vi "Balance Wheel.vi"() -> ()   [LabVIEW 2016]
uses:
  <vilib>/userdefined/High Color/nirio_resource_hc.ctl
  <vilib>/FPGAPlugInAG/myRIO-1900/niLvFpga_Open_myRIO-1900.vi
  <vilib>/rvi/interface/common/dynamic/niFpgaDynamicAddResources.vi
  <vilib>/Utility/error.llb/Error Cluster From Error Code.vi
  <vilib>/rvi/errors/niLvFpgaAdjustHostInterfaceError.vi
  <vilib>/FPGAPlugInAG/Dynamic/niLvFpga_Close_Dynamic.vi
  <vilib>/rvi/interface/nirviOpenFPGA/nirviOpenFPGA.xnode
  FPGA Bitfiles/BalanceWheel_FPGATarget_QuadratureEncode_czObzEe7hTA.lvbitx
  Quadrature Encoder FPGA.vi
  <vilib>/rvi/interface/nirviReadWriteControl/nirviReadWriteControl.xnode
  <vilib>/rvi/interface/nirviCloseFPGA/nirviCloseFPGA.xnode
  <vilib>/rvi/interface/Simulation/niFpgaSimulationCallBeginRW.vi
  NiFpgaLv.dll
panel:
  out "left":dbl=-0.003427734375000213 format="%#.1f"
  out "Rght":dbl=-0.003427734375000213 format="%#.1f"
  out "Desired Left Wheel Speed":dbl(knob)=-8.054739050568652e-09 scale=-5.0..5.0
  out "Displacement":dbl=0.9789672851562501
  out "Encoder Position 2":i32=45332
  in  "resource name":T1="RIO0"
  out "Encoder Position 1":i32=34865
  out "Right Wheel Speed":dbl(knob)=0.00244140625 scale=-5.0..5.0
  out "Left Wheel Speed":dbl(knob) scale=-5.0..5.0
  out "Speed of Car":dbl(knob)=0.001220703125 scale=-5.0..5.0
  out "Desired Right Wheel Speed":dbl(knob)=-8.054739050568652e-09 scale=-5.0..5.0
  out "Desired Speed of Car":dbl(knob)=-8.054739050568652e-09 scale=-5.0..5.0
  out "PID Right Wheel":dbl(knob)=0.20910621206179827 scale=-10.0..10.0
  out "PID Left Wheel":dbl(knob)=0.21032691478406132 scale=-10.0..10.0
  in  "KI (Right)":dbl=0.001
  in  "KP (Right)":dbl=0.5
  in  "KD (Right)":dbl
  in  "KI (Left)":dbl=0.001
  in  "KP (Left)":dbl=0.5
  in  "KD (Left)":dbl
  in  "stop":bool
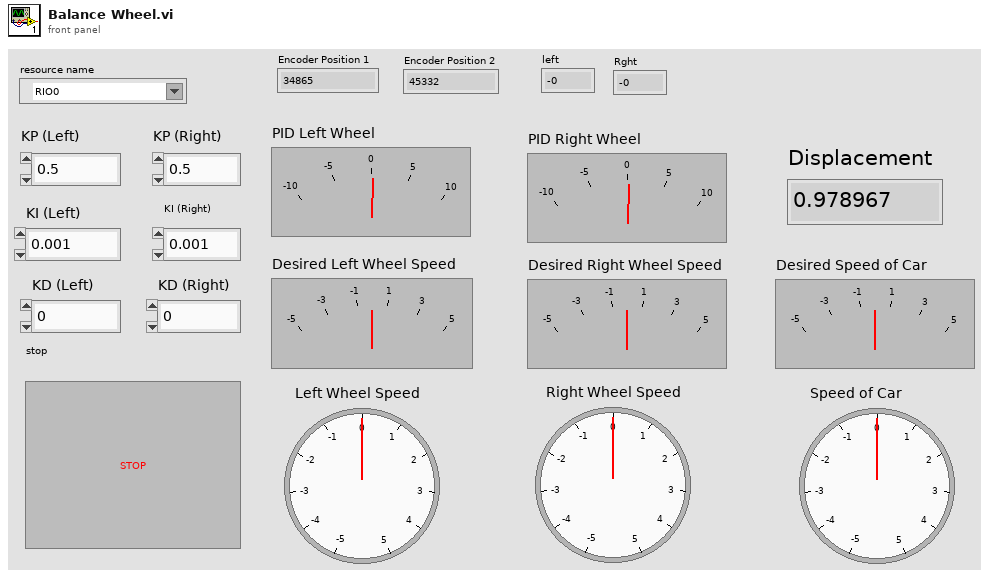
[diagram p1: front panel]
types:
  T1 = typedef "nirio_resource_hc.ctl" = tag
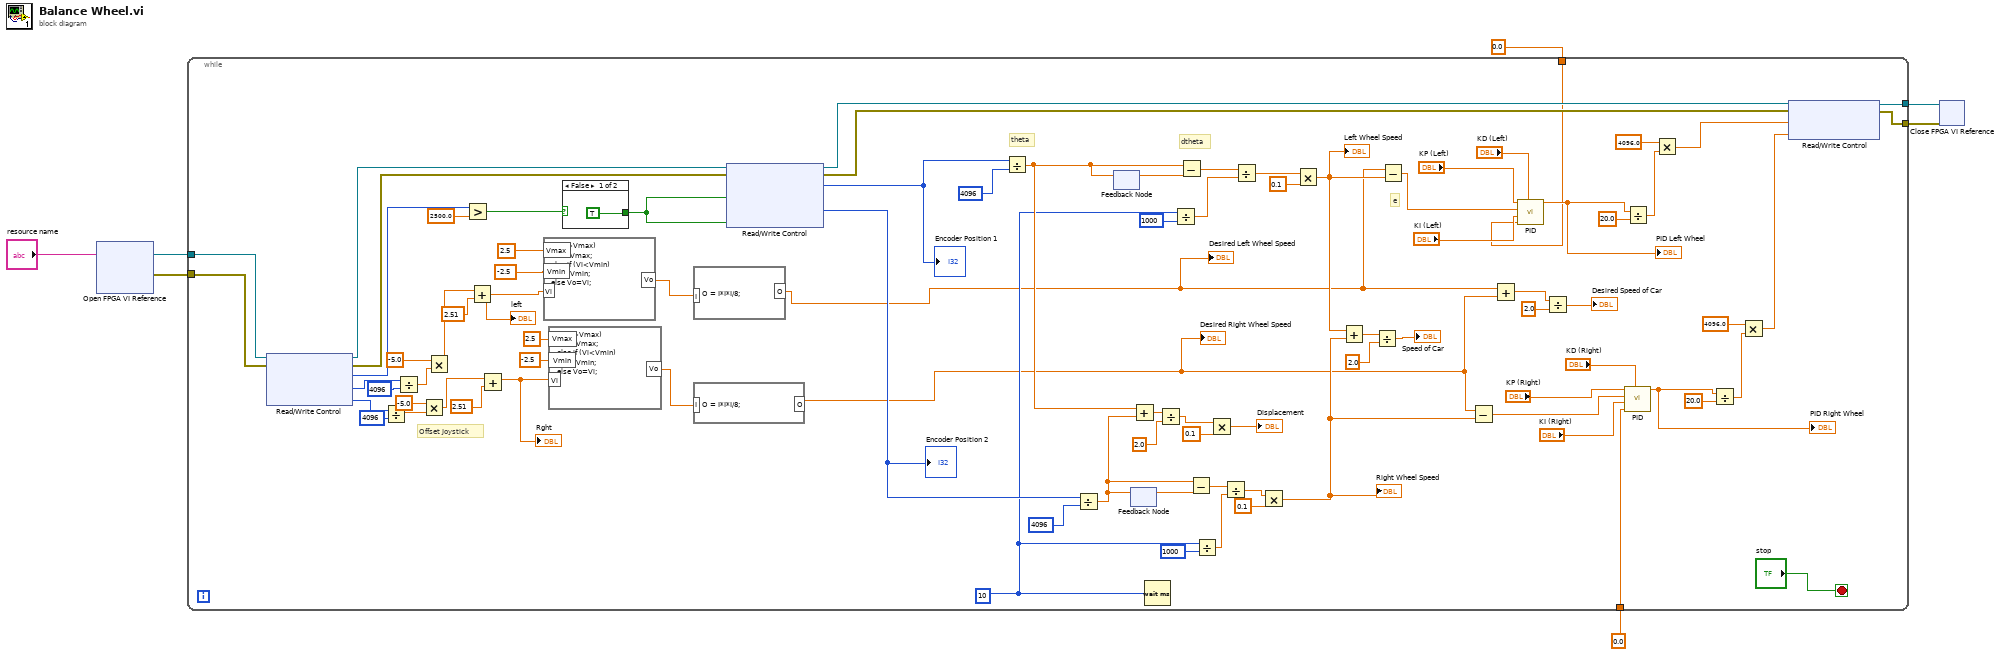
[diagram p0: block diagram]
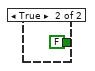
[diagram p2: hidden frame]
diagram:
  n1 = xnode "Open FPGA VI Reference"("resource name"="resource name") -> ("FPGA VI Reference Out"=w5:refnum<k20>, "error out"=w4:errorcluster)  [unwired: 1 in]
  n2 = while {
    tunnel: [w42] -> w7
    tunnel: [w41] -> w6
    tunnel: w5 -> [w11]
    tunnel: w4 -> [w10]
    tunnel: 0.0 ("Initial feedback in") -> [w9]
    tunnel: 0.0 ("Initial feedback in") -> [w8]
    stop <- "stop" stop-if-true
    w58 = u32 10 ("x")
    # "e"
    # "dtheta"
    # "theta"
    # "Offset Joystick"
    n3 = xnode "Read/Write Control"("FPGA VI Reference In"=w11, "error in"=w10) -> ("FPGA VI Reference Out"=w28:refnum<k20>, "error out"=w29:errorcluster, "ConnectorB/AI0"=w40:u16, "ConnectorB/AI1"=w39:u16, "ConnectorB/AI2"=w36:u16)
    n4 = Divide(x=w36, y=u16 4096) -> (x/y=w31:dbl)
    n5 = Divide(x=w39, y=u16 4096) -> (x/y=w35:dbl)
    n6 = Multiply(x=-5.0, y=w31) -> (x*y=w30:dbl)
    n7 = Multiply(x=-5.0, y=w35) -> (x*y=w33:dbl)
    n8 = Greater?(x=w40, y=2500.0) -> (0:w56:bool)
    n9 = Add(x=w33, y=2.51) -> (x+y=w47:dbl)
    "left" <- w47
    n10 = Add(x=w30, y=2.51) -> (x+y=w53:dbl)
    "Rght" <- w53
    n11 = formula code="if (Vi>Vmax)\nVo = Vmax;\nelse if (Vi<Vmin)\nVo = Vmin;\nelse Vo=Vi;"("Vi"=w47, "Vmin"=-2.5 ("input variable"), "Vmax"=2.5 ("input variable")) -> ("Vo"=w46:dbl)
    n12 = formula code="if (Vi>Vmax)\nVo = Vmax;\nelse if (Vi<Vmin)\nVo = Vmin;\nelse Vo=Vi;"("Vi"=w53, "Vmin"=-2.5 ("input variable"), "Vmax"=2.5 ("input variable")) -> ("Vo"=w50:dbl)
    n13 = case shown="False" w56 {
      tunnel: [TRUE ("Boolean 2") FALSE ("Boolean 2")] -> w45
      frame False {
      }
      frame True {
      }
    }
    n14 = formula code="O = I*I*I/8;"("I"=w46) -> ("O"=w13:dbl)
    "Desired Left Wheel Speed" <- w13
    n15 = formula code="O = I*I*I/8;"("I"=w50) -> ("O"=w12:dbl)
    "Desired Right Wheel Speed" <- w12
    n16 = xnode "Read/Write Control"("FPGA VI Reference In"=w28, "error in"=w29, "Reset - Quad 1"=w45, "Reset - Quad 2"=w45) -> ("FPGA VI Reference Out"=w44:refnum<k20>, "error out"=w43:errorcluster, "Encoder Position 1"=w75:i32, "Encoder Position 2"=w66:i32)
    "Encoder Position 1" <- w75
    "Encoder Position 2" <- w66
    n17 = Divide(x=w75, y=4096) -> (x/y=w65:dbl)
    n18 = Divide(x=w66, y=4096) -> (x/y=w64:dbl)
    n19 = feedback-in #1(w65) -> ()
    n20 = feedback #1() -> (w77:dbl)  [unwired: 1 in]
    n21 = feedback #2() -> (w69:dbl)  [unwired: 1 in]
    n22 = feedback-in #2(w64) -> ()
    n23 = Add(x=w65, y=w64) -> (x+y=w63:dbl)
    n24 = Wait (ms)(milliseconds to wait=w58) -> ()  [unwired: 1 out]
    n25 = Divide(x=w63, y=2.0) -> (x/y=w60:dbl)
    n26 = Divide(x=w58, y=u32 1000) -> (x/y=w82:dbl)
    n27 = Subtract(x=w65, y=w77) -> (x-y=w83:dbl)
    n28 = Subtract(x=w64, y=w69) -> (x-y=w74:dbl)
    n29 = Divide(x=w58, y=u32 1000) -> (x/y=w73:dbl)
    n30 = Multiply(x=w60, y=0.1) -> (x*y=→"Displacement":dbl)
    n31 = Divide(x=w74, y=w73) -> (x/y=w71:dbl)
    n32 = Divide(x=w83, y=w82) -> (x/y=w80:dbl)
    n33 = Multiply(x=w71, y=0.1) -> (x*y=w67:dbl)
    "Right Wheel Speed" <- w67
    n34 = Multiply(x=w80, y=0.1) -> (x*y=w79:dbl)
    "Left Wheel Speed" <- w79
    n35 = Add(x=w79, y=w67) -> (x+y=w89:dbl)
    n36 = Divide(x=w89, y=2.0) -> (x/y=→"Speed of Car":dbl)
    n37 = Subtract(x=w13, y=w79) -> (x-y=w18:dbl)
    n38 = Subtract(x=w12, y=w67) -> (x-y=w90:dbl)
    n39 = Add(x=w13, y=w12) -> (x+y=w86:dbl)
    n40 = call "PID.vi"("KD"="KD (Left)", "Initial feedback in"=w9, "KI"="KI (Left)", "Error in"=w18, "KP"="KP (Left)") -> ("PIDout"=w14:dbl)  [unwired: 6 in]
    "PID Left Wheel" <- w14
    n41 = Divide(x=w86, y=2.0) -> (x/y=→"Desired Speed of Car":dbl)
    n42 = call "PID.vi"("KD"="KD (Right)", "Initial feedback in"=w8, "KI"="KI (Right)", "Error in"=w90, "KP"="KP (Right)") -> ("PIDout"=w20:dbl)  [unwired: 6 in]
    "PID Right Wheel" <- w20
    n43 = Divide(x=w14, y=20.0) -> (x/y=w25:dbl)
    n44 = Multiply(x=4096.0, y=w25) -> (x*y=w26:dbl)
    n45 = Divide(x=w20, y=20.0) -> (x/y=w22:dbl)
    n46 = Multiply(x=4096.0, y=w22) -> (x*y=w19:dbl)
    n47 = xnode "Read/Write Control"("FPGA VI Reference In"=w44, "error in"=w43, "ConnectorC/AO0"=w26, "ConnectorC/AO1"=w19) -> ("FPGA VI Reference Out"=w42:refnum<k20>, "error out"=w41:errorcluster)
  }
  n48 = xnode "Close FPGA VI Reference"("FPGA VI Reference In"=w7, "error in"=w6) -> ()  [unwired: 1 out]
